vi "Normalize Path.vi"(1 "path":path) -> (0 "normalized path":path)   [LabVIEW 2021, in "MeasurementService Editor.lvlib"]
uses:
  MeasurementService Editor.lvlib
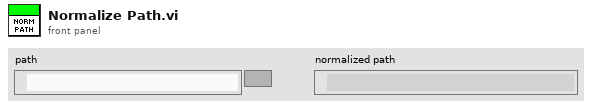
[diagram p1: front panel]
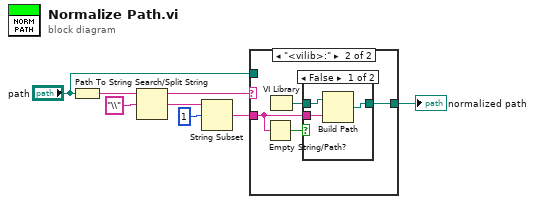
[diagram p0: block diagram]
diagram:
  n1 = Path To String(path="path") -> (string=w8:string)
  n2 = Search/Split String(string=w8, search string/char (-)="\\") -> (substring before match=w6:string, match + rest of string=w3:string)  [unwired: 1 in, 1 out]
  n3 = String Subset(string=w3, offset (0)=1) -> (substring=w4:string)  [unwired: 1 in]
  n4 = case shown="\"<vilib>:\"" w6 {
    tunnel: [w9 w12] -> w5
    tunnel: w4 -> [_ w11]
    tunnel: "path" -> [w9 _]
    frame Default {
    }
    frame "<vilib>:" {
      n5 = Empty String/Path?(string/path=w11) -> (empty?=w10:bool)
      n6 = VI Library() -> (path=w13:path)
      n7 = case shown="False" w10 {
        tunnel: w13 -> [w16 w17]
        tunnel: [w15 w17] -> w12
        tunnel: w11 -> [w14 _]
        frame False {
          n8 = Build Path(base path=w16, name or relative path=w14) -> (appended path=w15:path)
        }
        frame True {
        }
      }
    }
  }
  "normalized path" <- w5
